vi "shift register.vi"() -> ()   [LabVIEW 2020]
panel:
  out "Cluster":cluster{"Array 2":bool[], "Array 3":dbl[]}
  out "Array":bool[](array[boolean])
  out "Boolean":bool
  out "concatenated string":string
  out "Numeric":i32
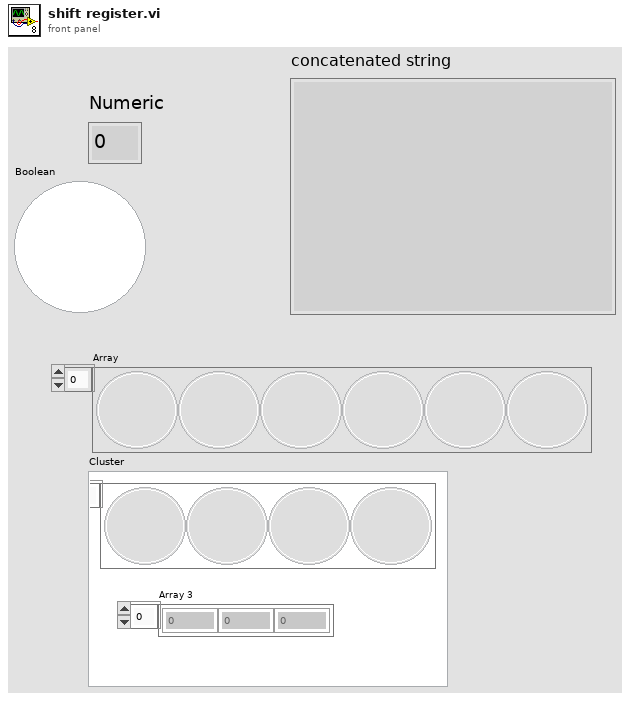
[diagram p1: front panel]
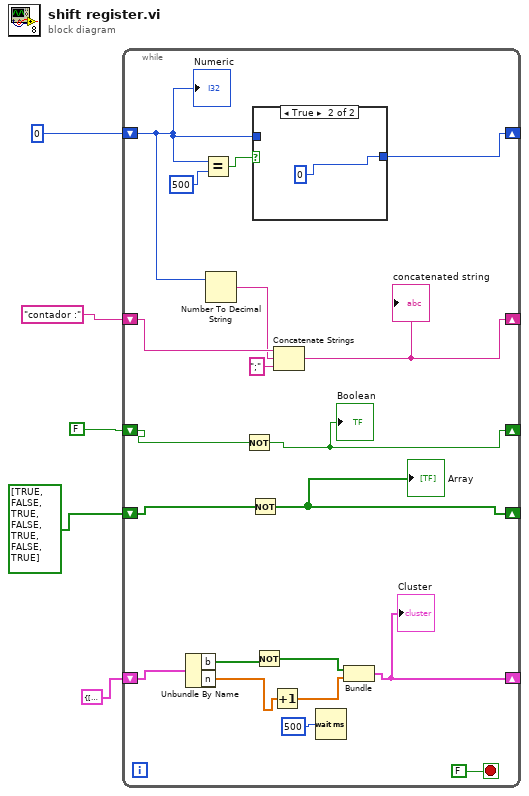
[diagram p0: block diagram]
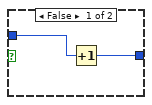
[diagram p2: hidden frame]
diagram:
  n1 = while {
    shift-right: [w22] -> _
    shift-left: 0 -> [w21]
    shift-right: [w17] -> _
    shift-left: "contador :" -> [w20]
    shift-right: [w15] -> _
    shift-left: FALSE -> [w16]
    shift-right: [w13] -> _
    shift-left: bool[] [TRUE, FALSE, TRUE, FALSE, TRUE, FALSE, TRUE] -> [w14]
    shift-right: [w7] -> _
    shift-left: cluster{"b":bool[], "n":dbl[]} {"b"=[FALSE, TRUE, FALSE, TRUE], "n"=[1.0, 2.0, 3.0]} -> [w12]
    stop <- FALSE stop-if-true
    n2 = Unbundle By Name(w12) -> ("b"=w11:bool[], "n"=w10:dbl[])
    n3 = Equal?(x=w21, y=500) -> (x = y?=w23:bool)
    n4 = Number To Decimal String(number=w21) -> (decimal integer string=w19:string)  [unwired: 1 in]
    n5 = Not(x=w16) -> (.not. x?=w15:bool)
    "Boolean" <- w15
    n6 = Not(x=w14) -> (.not. x?=w13:bool[])
    "Array" <- w13
    n7 = case shown="True" w23 {
      tunnel: w21 -> [w27 _]
      tunnel: [w26 0] -> w22
      frame False {
        n8 = Increment(x=w27) -> (x+1=w26:i32)
      }
      frame True {
      }
    }
    n9 = Not(x=w11) -> (.not. x?=w9:bool[])
    n10 = Increment(x=w10) -> (x+1=w8:dbl[])
    n11 = Concatenate Strings(w20, w19, ";" ("string")) -> (w17:string)
    "concatenated string" <- w17
    n12 = Wait (ms)(milliseconds to wait=u32 500) -> ()  [unwired: 1 out]
    n13 = Bundle(w9, w8) -> (w7:cluster{bool[], dbl[]})  [unwired: 1 in]
    "Cluster" <- w7
    "Numeric" <- w21
  }
